vi "Read ini.vi"(8 "error in (no error)":errorcluster, 10 "key":string="Reference Source", 11 "section":string="A") -> (0 "error out":errorcluster, 2 "Value":string[](array[string]))   [LabVIEW 2016]
uses:
  <vilib>/Utility/config.llb/Read Key (String).vi
  <vilib>/Utility/config.llb/NI_LVConfig.lvlib
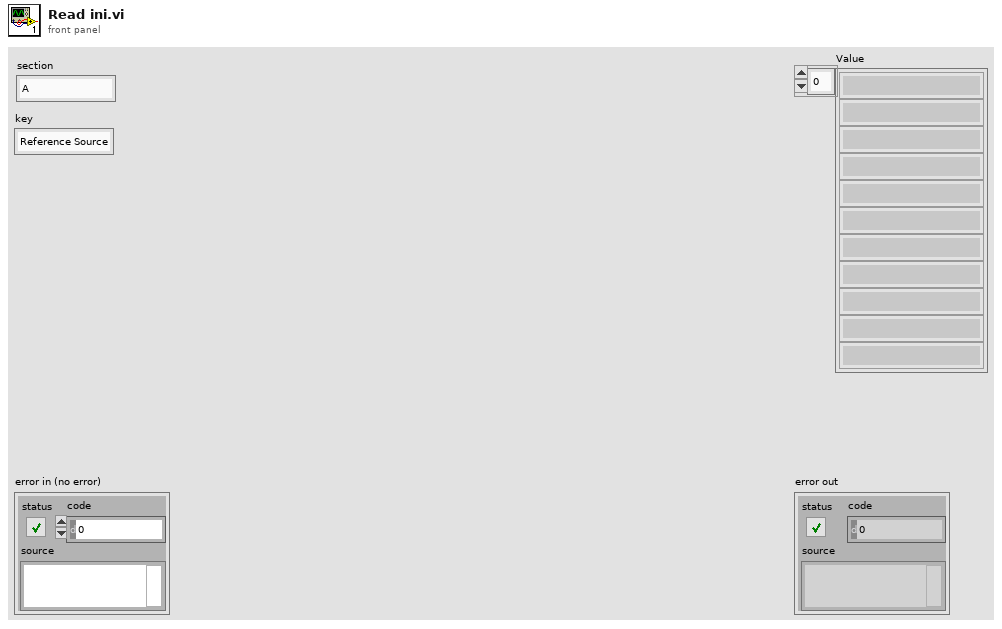
[diagram p1: front panel]
types:
  T1 = typedef "NI_LVConfig.lvlib/Config Data RefNum.ctl" = refnum<k1>
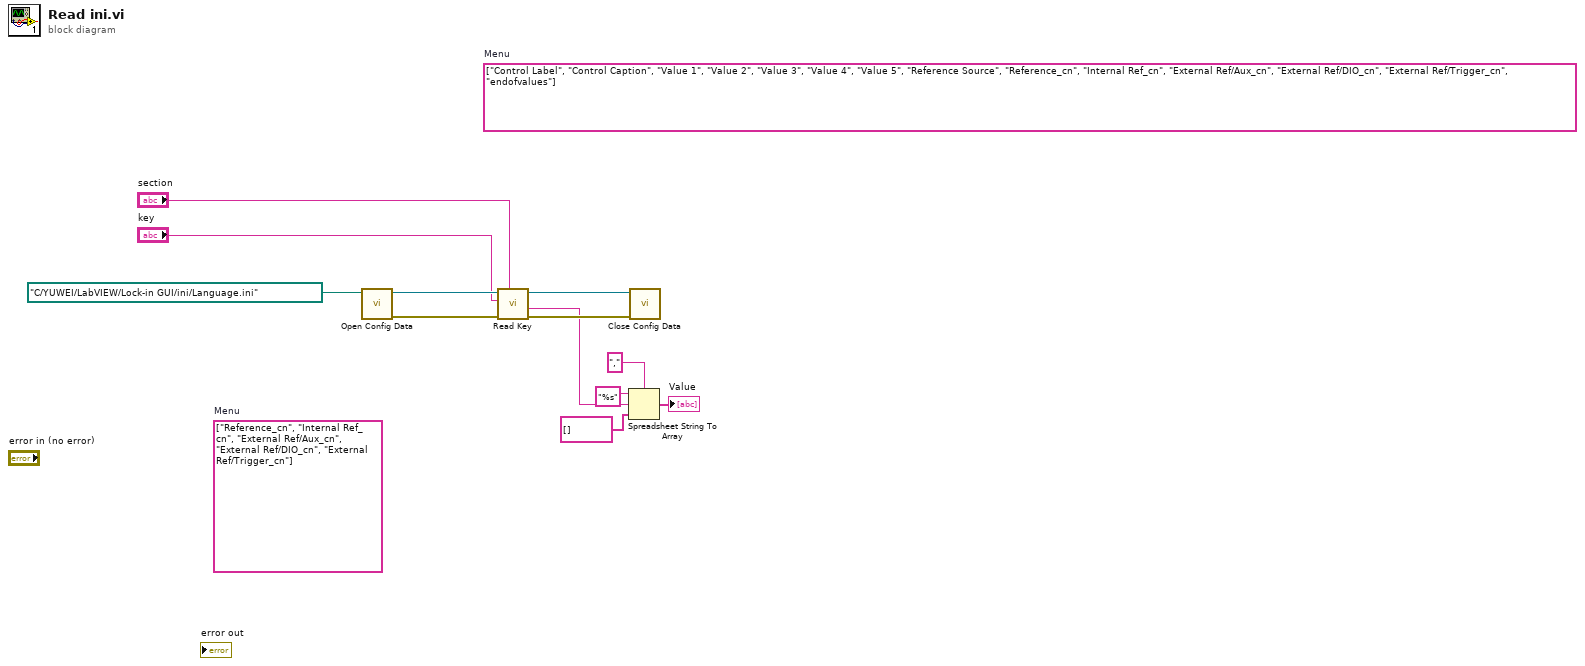
[diagram p0: block diagram]
diagram:
  (unwired) string[] ["Reference_cn", "Internal Ref_cn", "External Ref/Aux_cn", "External Ref/DIO_cn", "External Ref/Trigger_cn"]  # Menu
  (unwired) string[][] [["Control Label", "Control Caption", "Value 1", "Value 2", "Value 3", "Value 4", "Value 5"], ["Reference Source", "Reference_cn", "Internal Ref_cn", "External Ref/Aux_cn", "External Ref/DIO_cn", "External Ref/Trigger_cn", "endofvalues"]]  # Menu
  n1 = call <vilib>:"Open Config Data.vi"("configuration file path"=path "C:/YUWEI/LabVIEW/Lock-in GUI/ini/Language.ini") -> ("error out"=w11:errorcluster, "refnum"=w12:T1)  [unwired: 8 in, 1 out]
  n2 = call-poly <vilib>:"Read Key.vi"("section"="section", "error in (no error)"=w11, "key"="key", "refnum"=w12) -> ("error out"=w10:errorcluster, "value"=w3:string, "refnum out"=w9:T1)  [unwired: 4 in, 1 out]
  n3 = Spreadsheet String To Array(delimiter (Tab)=",", format string="%s", spreadsheet string=w3, array type (2D Dbl)=string[] []) -> (array=→"Value":string[])
  n4 = call <vilib>:"Close Config Data.vi"("error in (no error)"=w10, "refnum"=w9) -> ()  [unwired: 8 in, 2 out]
